vi "Get_Values.vi"(0 "reference in":refnum<class "Sig_AI.lvclass">) -> (6 "Data":T2, 13 "Scale":T1={"scale [EU/RAW]"=1.0, "offset [EU]"=0.0} {"offset [EU]" format="%0.2f"; "scale [EU/RAW]" format="%0.2f"})   [LabVIEW 2019, in "Sig_AI.lvclass"]
uses:
  Sig_AI.lvclass
  TypeDef/AI_Data.ctl
  TypeDef/Config_Scale.ctl
  Sig_AI.lvclass/Sig_AI.ctl
  AnalogComparator_class/AnalogComparator.lvclass/AnalogComparator.ctl
  AnalogComparator_class/AnalogComparator.lvclass
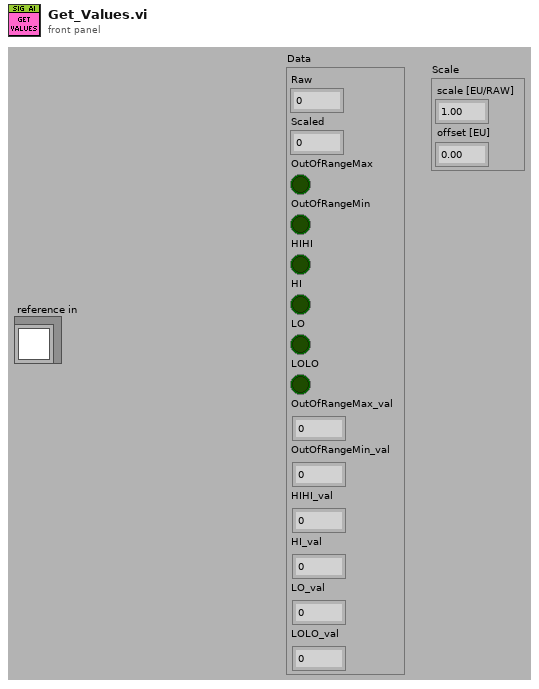
[diagram p1: front panel]
types:
  T1 = typedef "Config_Scale.ctl" = cluster{"scale [EU/RAW]":dbl, "offset [EU]":dbl}
  T2 = typedef "AI_Data.ctl" = cluster{"Raw":dbl, "Scaled":dbl, "OutOfRangeMax":bool, "OutOfRangeMin":bool, "HIHI":bool, "HI":bool, "LO":bool, "LOLO":bool, "OutOfRangeMax_val":dbl, "OutOfRangeMin_val":dbl, "HIHI_val":dbl, "HI_val":dbl, "LO_val":dbl, "LOLO_val":dbl}
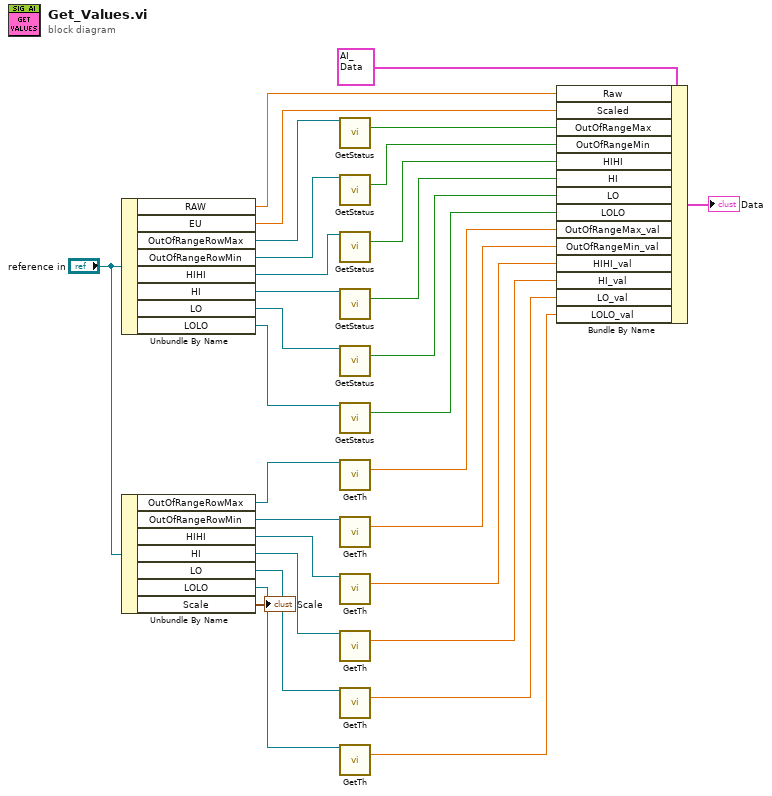
[diagram p0: block diagram]
diagram:
  n1 = Unbundle By Name("reference in") -> ("RAW"=w29:dbl, "EU"=w28:dbl, "OutOfRangeRowMax"=w27:refnum<class "AnalogComparator.lvclass">, "OutOfRangeRowMin"=w25:refnum<class "AnalogComparator.lvclass">, "HIHI"=w24:refnum<class "AnalogComparator.lvclass">, "HI"=w23:refnum<class "AnalogComparator.lvclass">, "LO"=w22:refnum<class "AnalogComparator.lvclass">, "LOLO"=w21:refnum<class "AnalogComparator.lvclass">)
  n2 = Unbundle By Name("reference in") -> ("OutOfRangeRowMax"=w13:refnum<class "AnalogComparator.lvclass">, "OutOfRangeRowMin"=w12:refnum<class "AnalogComparator.lvclass">, "HIHI"=w11:refnum<class "AnalogComparator.lvclass">, "HI"=w10:refnum<class "AnalogComparator.lvclass">, "LO"=w9:refnum<class "AnalogComparator.lvclass">, "LOLO"=w8:refnum<class "AnalogComparator.lvclass">, "Scale"=→"Scale":T1)
  n3 = call "GetStatus.vi"("class data in"=w27) -> ("Status"=w26:bool)  [unwired: 14 in]
  n4 = call "GetStatus.vi"("class data in"=w25) -> ("Status"=w20:bool)  [unwired: 14 in]
  n5 = call "GetStatus.vi"("class data in"=w24) -> ("Status"=w19:bool)  [unwired: 14 in]
  n6 = call "GetStatus.vi"("class data in"=w23) -> ("Status"=w18:bool)  [unwired: 14 in]
  n7 = call "GetStatus.vi"("class data in"=w22) -> ("Status"=w17:bool)  [unwired: 14 in]
  n8 = call "GetStatus.vi"("class data in"=w21) -> ("Status"=w16:bool)  [unwired: 14 in]
  n9 = call "GetTh.vi"("class data in"=w13) -> ("configAnalogComp.Threshold"=w7:dbl)  [unwired: 14 in]
  n10 = call "GetTh.vi"("class data in"=w12) -> ("configAnalogComp.Threshold"=w6:dbl)  [unwired: 14 in]
  n11 = call "GetTh.vi"("class data in"=w11) -> ("configAnalogComp.Threshold"=w5:dbl)  [unwired: 14 in]
  n12 = call "GetTh.vi"("class data in"=w10) -> ("configAnalogComp.Threshold"=w4:dbl)  [unwired: 14 in]
  n13 = call "GetTh.vi"("class data in"=w9) -> ("configAnalogComp.Threshold"=w3:dbl)  [unwired: 14 in]
  n14 = call "GetTh.vi"("class data in"=w8) -> ("configAnalogComp.Threshold"=w2:dbl)  [unwired: 14 in]
  n15 = Bundle By Name(cluster=T2 {"Raw"=0.0, "Scaled"=0.0, "OutOfRangeMax"=FALSE, "OutOfRangeMin"=FALSE, "HIHI"=FALSE, "HI"=FALSE, "LO"=FALSE, "LOLO"=FALSE, "OutOfRangeMax_val"=0.0, "OutOfRangeMin_val"=0.0, "HIHI_val"=0.0, "HI_val"=0.0, "LO_val"=0.0, "LOLO_val"=0.0} ("AI_Data"), "Raw"=w29, "Scaled"=w28, "OutOfRangeMax"=w26, "OutOfRangeMin"=w20, "HIHI"=w19, "HI"=w18, "LO"=w17, "LOLO"=w16, "OutOfRangeMax_val"=w7, "OutOfRangeMin_val"=w6, "HIHI_val"=w5, "HI_val"=w4, "LO_val"=w3, "LOLO_val"=w2) -> (→"Data":T2)
